vi "HOL_SWERVE_ODOM_REL_FGV.vi"(9 "in SWERVE_DRIVE_ODOMETRY":T1={"POSE"={"TRANSLATION"={"X"=0.0, "Y"=0.0}, "ROTATION"={"VALUE"=0.0, "COS"=1.0, "SIN"=0.0}}, "GyroOffset"={"VALUE"=0.0, "COS"=1.0, "SIN"=0.0}, "PreviousAngle"={"VALUE"=0.0, "COS"=1.0, "SIN"=0.0}, "PrevModulePositions"=[], "NumModules"=0} {"PrevModulePositions"."Angle"."SIN" format="%13.4f"; "PrevModulePositions"."Angle"."COS" format="%13.4f"; "PrevModulePositions"."Angle"."VALUE" format="%13.4f"; "PreviousAngle"."SIN" format="%13.4f"; "PreviousAngle"."COS" format="%13.4f"; "PreviousAngle"."VALUE" format="%13.4f"; "GyroOffset"."SIN" format="%13.4f"; "GyroOffset"."COS" format="%13.4f"; "GyroOffset"."VALUE" format="%13.4f"; "POSE"."ROTATION"."SIN" format="%13.4f"; "POSE"."ROTATION"."COS" format="%13.4f"; "POSE"."ROTATION"."VALUE" format="%13.4f"; "POSE"."TRANSLATION"."Y" format="%14.3f"; "POSE"."TRANSLATION"."X" format="%14.3f"}, 11 "WRITE":bool) -> (1 "out SWERVE_DRIVE_ODOMETRY":T1={"POSE"={"TRANSLATION"={"X"=0.0, "Y"=0.0}, "ROTATION"={"VALUE"=0.0, "COS"=1.0, "SIN"=0.0}}, "GyroOffset"={"VALUE"=0.0, "COS"=1.0, "SIN"=0.0}, "PreviousAngle"={"VALUE"=0.0, "COS"=1.0, "SIN"=0.0}, "PrevModulePositions"=[], "NumModules"=0} {"PrevModulePositions"."Angle"."SIN" format="%13.4f"; "PrevModulePositions"."Angle"."COS" format="%13.4f"; "PrevModulePositions"."Angle"."VALUE" format="%13.4f"; "PreviousAngle"."SIN" format="%13.4f"; "PreviousAngle"."COS" format="%13.4f"; "PreviousAngle"."VALUE" format="%13.4f"; "GyroOffset"."SIN" format="%13.4f"; "GyroOffset"."COS" format="%13.4f"; "GyroOffset"."VALUE" format="%13.4f"; "POSE"."ROTATION"."SIN" format="%13.4f"; "POSE"."ROTATION"."COS" format="%13.4f"; "POSE"."ROTATION"."VALUE" format="%13.4f"; "POSE"."TRANSLATION"."Y" format="%14.3f"; "POSE"."TRANSLATION"."X" format="%14.3f"})   [LabVIEW 2019]
uses:
  <vilib>/Rock Robotics/WPI/ThirdParty/JAS_Junk/TrajLib/TypeDef/SWERVE_DRIVE_ODOMETRY.ctl
  <vilib>/Rock Robotics/WPI/ThirdParty/JAS_Junk/TrajLib/TypeDef/POSE2D.ctl
  <vilib>/Rock Robotics/WPI/ThirdParty/JAS_Junk/TrajLib/TypeDef/TRANSLATION2D.ctl
  <vilib>/Rock Robotics/WPI/ThirdParty/JAS_Junk/TrajLib/TypeDef/ROTATION2D.ctl
  <vilib>/Rock Robotics/WPI/ThirdParty/JAS_Junk/TrajLib/TypeDef/SWERVE_DRIVE_MODULE_POSITION.ctl
  <vilib>/Rock Robotics/WPI/ThirdParty/JAS_Junk/TrajLib/Trajectory_Library.lvlib
panel:
  # "This is purposefully \n\nNOT re-entrant."
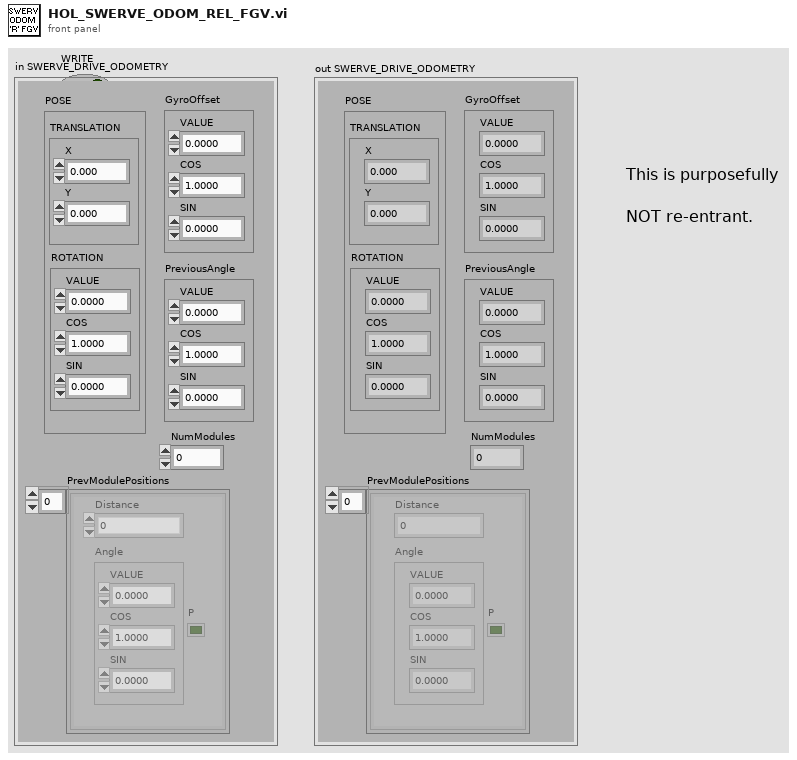
[diagram p1: front panel]
types:
  T1 = typedef "Trajectory_Library.lvlib/SWERVE_DRIVE_ODOMETRY.ctl" = cluster{"POSE":T2, "GyroOffset":T4, "PreviousAngle":T4, "PrevModulePositions":T5[], "NumModules":i32}
  T2 = typedef "Trajectory_Library.lvlib/POSE2D.ctl" = cluster{"TRANSLATION":T3, "ROTATION":T4}
  T3 = typedef "Trajectory_Library.lvlib/TRANSLATION2D.ctl" = cluster{"X":dbl, "Y":dbl}
  T4 = typedef "Trajectory_Library.lvlib/ROTATION2D.ctl" = cluster{"VALUE":dbl, "COS":dbl, "SIN":dbl}
  T5 = typedef "Trajectory_Library.lvlib/SWERVE_DRIVE_MODULE_POSITION.ctl" = cluster{"Distance":dbl, "Angle":T4, "P":bool}
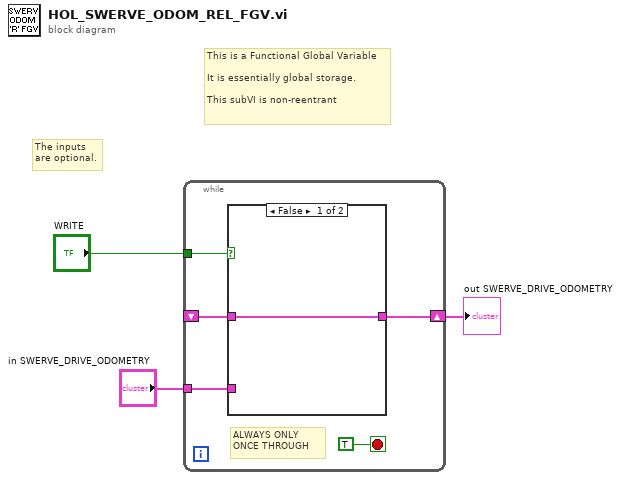
[diagram p0: block diagram]
diagram:
  # "The inputs \nare optional."
  # "This is a Functional Global Variable\n\nIt is essentially global storage.\n\nThis subVI is non-reentrant"
  n1 = while {
    shift-right: [w6] -> w1
    shift-left: _ -> [w4]
    tunnel: "WRITE" -> [w7]
    tunnel: "in SWERVE_DRIVE_ODOMETRY" -> [w5]
    stop <- TRUE stop-if-true
    # "ALWAYS ONLY\nONCE THROUGH"
    n2 = case shown="False" w7 {
      tunnel: [w9 w10] -> w6
      tunnel: w5 -> [_ w10]
      tunnel: w4 -> [w9 _]
      frame False {
      }
      frame True {
      }
    }
  }
  "out SWERVE_DRIVE_ODOMETRY" <- w1
